vi "Read PGPASS.vi"(8 "error in":errorcluster) -> (0 "error out":errorcluster, 1 "Connection Information":T1, 2 "connection string":string)   [LabVIEW 2016, in "PQ Support.lvlib"]
uses:
  PQ Support.lvlib
  Connection Information.ctl
  <vilib>/Utility/sysdir.llb/System Directory Type.ctl
  <userlib>/_OpenG.lib/file/file.llb/File Exists - Scalar__ogtk.vi
  Connection/PQ Connection.lvclass
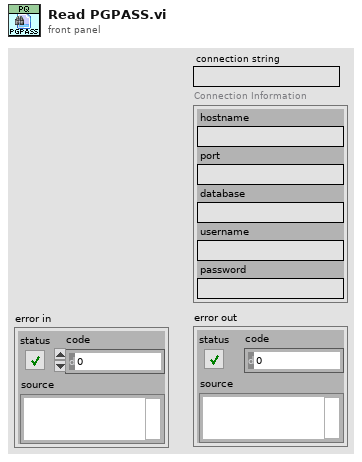
[diagram p1: front panel]
types:
  T1 = typedef "PQ Connection.lvclass/Connection Information.ctl" = cluster{"hostname":string, "port":string, "database":string, "username":string, "password":string}
  T2 = typedef "System Directory Type.ctl" = i32
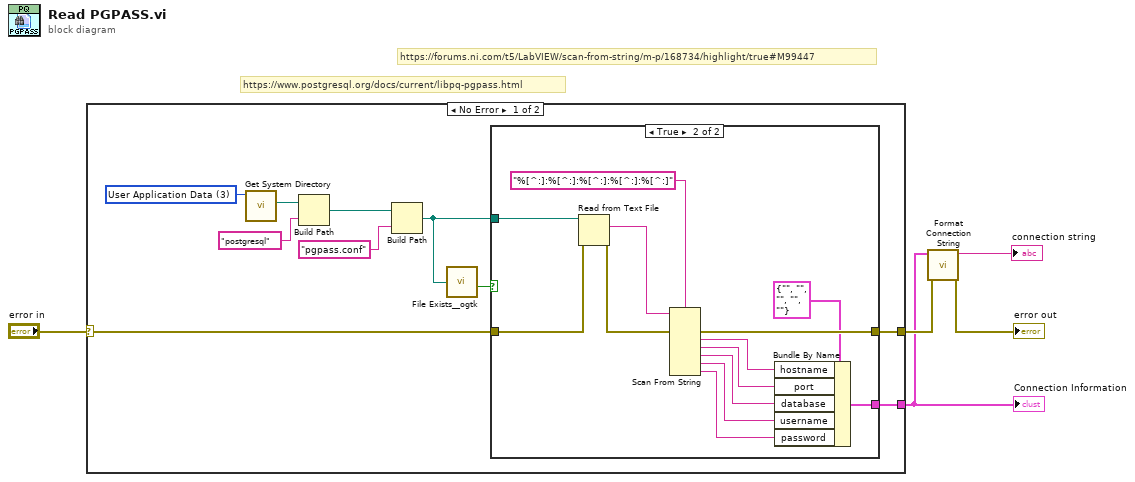
[diagram p0: block diagram]
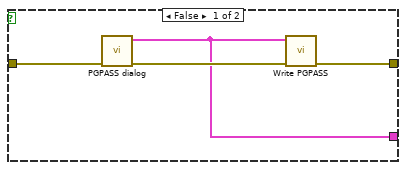
[diagram p2: hidden frame]
diagram:
  # "https://forums.ni.com/t5/LabVIEW/scan-from-string/m-p/168734/highlight/true#M99447"
  # "https://www.postgresql.org/docs/current/libpq-pgpass.html"
  n1 = case shown="No Error" "error in" {
    selector: "error in" -> [w9 w33]
    tunnel: [w10 w33] -> w4
    tunnel: [w8 _] -> w2
    frame No Error {
      w15 = T2 3 items=["User Home"=0, "User Desktop"=1, "User Documents"=2, "User Application Data"=3, "User Preferences"=4, "User Temporary"=5, "Public Documents"=6, "Public Application Data"=7, "Public Preferences"=8, "Public Cache"=13, "System Core Libraries"=9, "System Installed Libraries"=10, "Application Files"=11, "Boot Volume Root"=12] ("system directory type")
      n2 = call <vilib>:"Get System Directory.vi"("system directory type"=w15) -> ("system directory"=w14:path)  [unwired: 10 in]
      n3 = Build Path(base path=w14, name or relative path="postgresql") -> (appended path=w12:path)
      n4 = Build Path(base path=w12, name or relative path="pgpass.conf") -> (appended path=w7:path)
      n5 = call-poly <userlib>:"File Exists__ogtk.vi"("file path"=w7) -> ("exists"=w6:bool)  [unwired: 6 in, 1 out]
      n6 = case shown="True" w6 {
        tunnel: [w19 w31] -> w10
        tunnel: w9 -> [w17 w30]
        tunnel: [w16 w22] -> w8
        tunnel: w7 -> [_ w20]
        frame False {
          n7 = call "PGPASS dialog.vi"("error in (no error)"=w17) -> ("error out"=w18:errorcluster, "Connection Information"=w16:T1)  [unwired: 9 in]
          n8 = call "Write PGPASS.vi"("error in"=w18, "Connection Information"=w16) -> ("error out"=w19:errorcluster)  [unwired: 9 in]
        }
        frame True {
          n9 = Read from Text File(file (use dialog)=w20, error in=w30) -> (text=w29:string, error out=w21:errorcluster)  [unwired: 2 in, 2 out]
          n10 = Scan From String(format string="%[^:]:%[^:]:%[^:]:%[^:]:%[^:]", input string=w29, error in=w21) -> (error out=w31:errorcluster, output 1=w27:string, output 2=w26:string, output 3=w25:string, output 4=w24:string, output 5=w23:string)  [unwired: 6 in, 2 out]
          n11 = Bundle By Name(cluster=T1 {"hostname"="", "port"="", "database"="", "username"="", "password"=""} ("Connection Information"), "hostname"=w27, "port"=w26, "database"=w25, "username"=w24, "password"=w23) -> (w22:T1)
        }
      }
    }
    frame Error {
    }
  }
  "Connection Information" <- w2
  n12 = call "Format Connection String.vi"("error in"=w4, "Connection Information"=w2) -> ("error out"=→"error out":errorcluster, "connection string"=→"connection string":string)  [unwired: 8 in]
